vi "Variant to Data String.vi"(10 "error in (no error)":errorcluster, 11 "Data":variant) -> (2 "error out":errorcluster, 3 "string":string)   [LabVIEW 2020, in "RxnRover.lvlib"]
uses:
  RxnRover.lvlib
  <vilib>/Utility/Data Type/NI_Data Type.lvlib
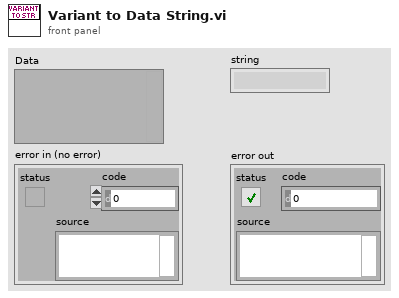
[diagram p1: front panel]
types:
  T1 = typedef "NI_Data Type.lvlib/Data Type.ctl" = enum8{"Invalid Type", "Void", "I8", "I16", "I32", "I64", "U8", "U16", "U32", "U64", "Single Float", "Double Float", "Extended Float", "Single Complex", "Double Complex", "Extended Complex", "Enum U8", "Enum U16", "Enum U32", "Enum U64", "Single Float With Unit", "Double Float With Unit", "Extended Float With Unit", "Single Complex with Unit", "Double Complex with Unit", "Extended Complex with Unit", "Boolean", "String", "Path", "Picture", "Tag", "Array", "Cluster", "Variant", "LV Variant", "Waveform", "Timestamp", "Digital Waveform", "Digital Data", "ExpressData", "Refnum", "External Data", "VI", "Poly VI", "LabVIEW Class Instance", "Fixed Point", "Set Collection", "Map Collection"}
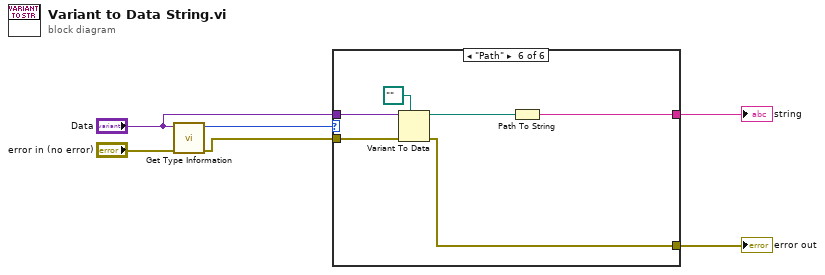
[diagram p0: block diagram]
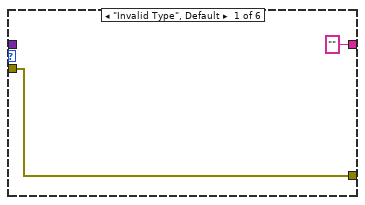
[diagram p2: hidden frame]
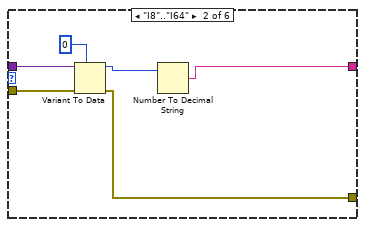
[diagram p3: hidden frame]
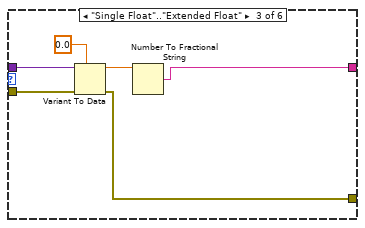
[diagram p4: hidden frame]
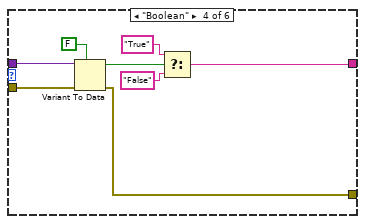
[diagram p5: hidden frame]
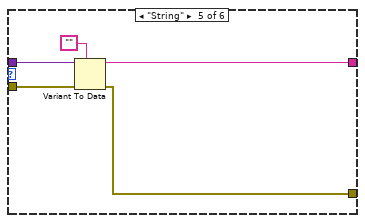
[diagram p6: hidden frame]
diagram:
  n1 = call <vilib>:"Get Type Information.vi"("error in (no error)"="error in (no error)", "variant"="Data") -> ("error out"=w4:errorcluster, "type"=w6:T1)  [unwired: 5 in, 3 out]
  n2 = case shown="\"Path\"" w6 {
    tunnel: "Data" -> [_ w14 w20 w28 w33 w39]
    tunnel: w4 -> [w7 w13 w19 w27 w32 w38]
    tunnel: [w7 w12 w18 w26 w31 w37] -> w3
    tunnel: ["" w9 w15 w21 w29 w34] -> w2
    frame "Invalid Type", Default {
    }
    frame "I8".."I64" {
      n3 = Variant To Data(error in=w13, type=0, Variant=w14) -> (data=w10:i32, error out=w12:errorcluster)
      n4 = Number To Decimal String(number=w10) -> (decimal integer string=w9:string)  [unwired: 1 in]
    }
    frame "Single Float".."Extended Float" {
      n5 = Variant To Data(error in=w19, type=0.0, Variant=w20) -> (data=w16:dbl, error out=w18:errorcluster)
      n6 = Number To Fractional String(number=w16) -> (F-format string=w15:string)  [unwired: 3 in]
    }
    frame "Boolean" {
      n7 = Variant To Data(error in=w27, type=FALSE, Variant=w28) -> (data=w24:bool, error out=w26:errorcluster)
      n8 = Select(t="True", s=w24, f="False") -> (s? t:f=w21:string)
    }
    frame "String" {
      n9 = Variant To Data(error in=w32, type="", Variant=w33) -> (data=w29:string, error out=w31:errorcluster)
    }
    frame "Path" {
      n10 = Variant To Data(error in=w38, type=path "", Variant=w39) -> (data=w35:path, error out=w37:errorcluster)
      n11 = Path To String(path=w35) -> (string=w34:string)
    }
  }
  "string" <- w2
  "error out" <- w3
